vi "Lockin Read Settings.vi"(8 "errorIN":errorcluster caption="Error") -> (0 "errorOUT":errorcluster caption="Error", 3 "lockinsettings":T2(array[cluster]))   [LabVIEW 2017, in "SR830.lvlib"]
uses:
  SR830.lvlib
  Global/GPIB Numbers.vi
panel:
  out "chan2display":T1(ring)
  out "chan1display":enum16{"X", "R", "X Noise", "Aux 1", "Aux 2"}(ring)
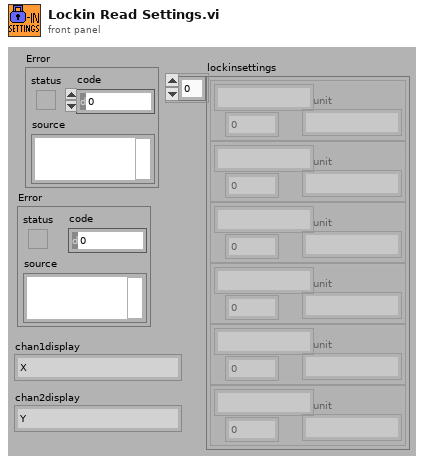
[diagram p1: front panel]
types:
  T1 = enum16{"Y", "Theta", "Y Noise", "Aux 3", "Aux 4"}
  T2 = cluster{"name":string, "value":dbl, "unit":string}[]
  T3 = typedef "GPIB Type Def.ctl" = cluster{"Name":string, "bus":dbl, "GPIB":dbl, "GPIB as string":string, "byte":i32, "VISA Resource Name":refnum<visa-resource-name>}
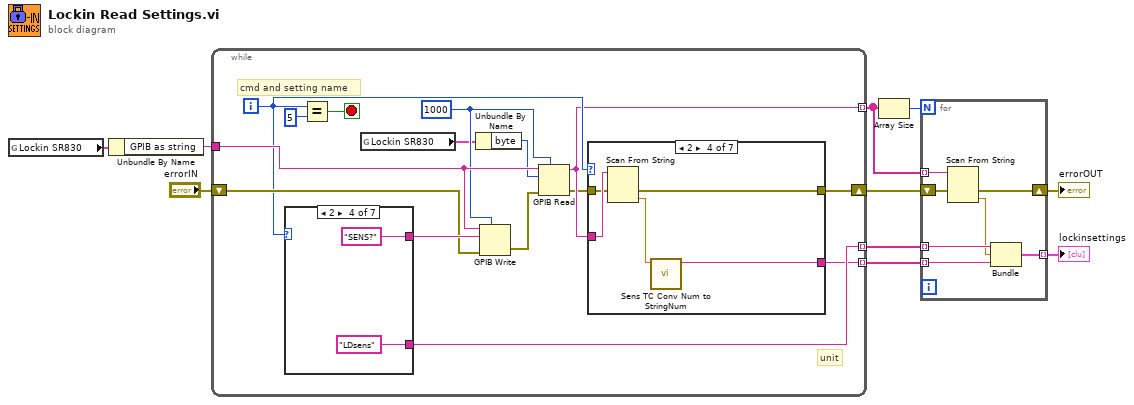
[diagram p0: block diagram]
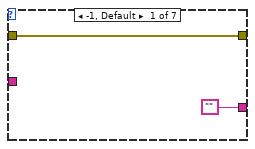
[diagram p2: hidden frame]
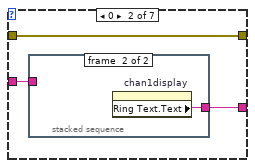
[diagram p3: hidden frame]
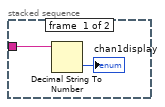
[diagram p4: hidden frame]
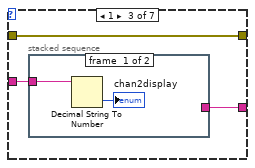
[diagram p5: hidden frame]
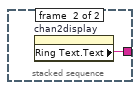
[diagram p6: hidden frame]
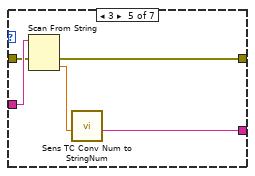
[diagram p7: hidden frame]
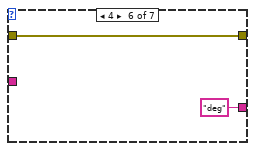
[diagram p8: hidden frame]
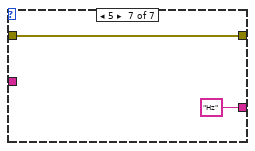
[diagram p9: hidden frame]
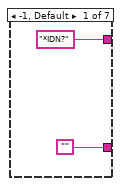
[diagram p10: hidden frame]
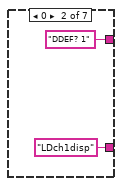
[diagram p11: hidden frame]
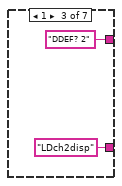
[diagram p12: hidden frame]
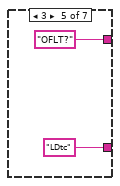
[diagram p13: hidden frame]
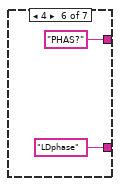
[diagram p14: hidden frame]
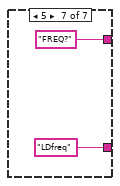
[diagram p15: hidden frame]
diagram:
  n1 = global read "GPIB Numbers.vi" "Lockin SR830"() -> (w10:T3)
  n2 = Unbundle By Name(w10) -> ("GPIB as string"=w9:string)
  n3 = while {
    tunnel: w9 -> [w23]
    shift-right: [w11] -> w2
    shift-left: "errorIN" -> [w19]
    tunnel: [w16] -> w6 mode=indexing
    tunnel: [w18] -> w5 mode=indexing
    tunnel: [w15] -> w4 mode=indexing
    i -> [w17]
    stop <- w25 stop-if-true
    w22 = 1000
    # "cmd and setting name"
    # "unit"
    n4 = case shown="2" w17 {
      tunnel: ["*IDN?" "DDEF? 1" "DDEF? 2" "SENS?" "OFLT?" "PHAS?" "FREQ?"] -> w21
      tunnel: ["" "LDch1disp" "LDch2disp" "LDsens" "LDtc" "LDphase" "LDfreq"] -> w18
      frame -1, Default {
      }
      frame 0 {
      }
      frame 1 {
      }
      frame 2 {
      }
      frame 3 {
      }
      frame 4 {
      }
      frame 5 {
      }
    }
    n5 = Equal?(x=w17, y=5) -> (x = y?=w25:bool)
    n6 = global read "GPIB Numbers.vi" "Lockin SR830"() -> (w14:T3)
    n7 = Unbundle By Name(w14) -> ("byte"=w13:i32)
    n8 = GPIB Write(0:w23, 1:w21, 3:w19, 4:w22) -> (6:w20:errorcluster)  [unwired: 2 out]
    n9 = GPIB Read(0:w23, 1:w13, 3:w20, 4:w22) -> (5:w16:string, 7:w12:errorcluster)  [unwired: 2 out]
    n10 = case shown="2" w17 {
      tunnel: w16 -> [_ w30 w36 w44 w49 _ _]
      tunnel: ["" w29 w35 w42 w48 "deg" "Hz"] -> w15
      tunnel: w12 -> [w26 w28 w34 w41 w46 w50 w52]
      tunnel: [w26 w28 w34 w40 w45 w50 w52] -> w11
      frame -1, Default {
      }
      frame 0 {
        n11 = stacked-sequence {
          tunnel: w30 -> [w32 _]
          tunnel: [_ w33] -> w29
          frame #0 {
            n12 = Decimal String To Number(string=w32) -> (number=→"chan1display":i32)  [unwired: 3 out]
          }
          frame #1 {
            n13 = property on="chan1display" class="Enum (strict)"() -> ("Ring Text.Text"=w33:string)  [unwired: 2 in, 2 out]
          }
        }
      }
      frame 1 {
        n14 = stacked-sequence {
          tunnel: w36 -> [w38 _]
          tunnel: [_ w39] -> w35
          frame #0 {
            n15 = Decimal String To Number(string=w38) -> (number=→"chan2display":i32)  [unwired: 3 out]
          }
          frame #1 {
            n16 = property on="chan2display" class="Enum (strict)"() -> ("Ring Text.Text"=w39:string)  [unwired: 2 in, 2 out]
          }
        }
      }
      frame 2 {
        n17 = Scan From String(input string=w44, error in=w41) -> (error out=w40:errorcluster, output 1=w43:dbl)  [unwired: 2 in, 3 out]
        n18 = call "Sens TC Conv Num to StringNum.vi"("sens"=w43) -> ("sensstring"=w42:string)  [unwired: 1 in, 9 out]
      }
      frame 3 {
        n19 = Scan From String(input string=w49, error in=w46) -> (error out=w45:errorcluster, output 1=w47:dbl)  [unwired: 2 in, 3 out]
        n20 = call "Sens TC Conv Num to StringNum.vi"("timeconst"=w47) -> ("tcstring"=w48:string)  [unwired: 1 in, 9 out]
      }
      frame 4 {
      }
      frame 5 {
      }
    }
  }
  n21 = Array Size(array=w6) -> (size(s)=w7:i32)
  n22 = for {
    N: w7 -> [_]
    tunnel: w6 -> [w74] mode=indexing
    tunnel: w5 -> [w73] mode=indexing
    tunnel: [w71] -> w3 mode=indexing
    tunnel: w4 -> [w70] mode=indexing
    shift-right: [w68] -> w1
    shift-left: w2 -> [w69]
    n23 = Scan From String(input string=w74, error in=w69) -> (error out=w68:errorcluster, output 1=w72:dbl)  [unwired: 2 in, 3 out]
    n24 = Bundle(w73, w72, "tcstring"=w70) -> (w71:cluster{string, dbl, "tcstring":string})  [unwired: 1 out]
  }
  "errorOUT" <- w1
  "lockinsettings" <- w3
